vi "PCE-info.vi"(0 "connection ID":refnum<k5>, 11 "error in":errorcluster) -> (4 "connection ID dup":refnum<k5>, 13 "Data Cluster":T1 {"Rotateur" format="%.2f"; "Dome" format="%.2f"; "Focus" format="%.2f"; "Année" format="%.2f"; "Temps Universel" format="%<%H:%M:%S%0u>t"; "Temps Sidéral" format="%<%H:%M:%S%0u>t"; "Masse d'air" format="%.2f"; "Epoque" format="%.2f"; "DEC" format="%<%H:%M:%S%0u>t"; "RA" format="%<%H:%M:%S%0u>t"; "HA" format="%<%H:%M:%S%0u>t"}, 15 "error out":errorcluster)   [LabVIEW 2011]
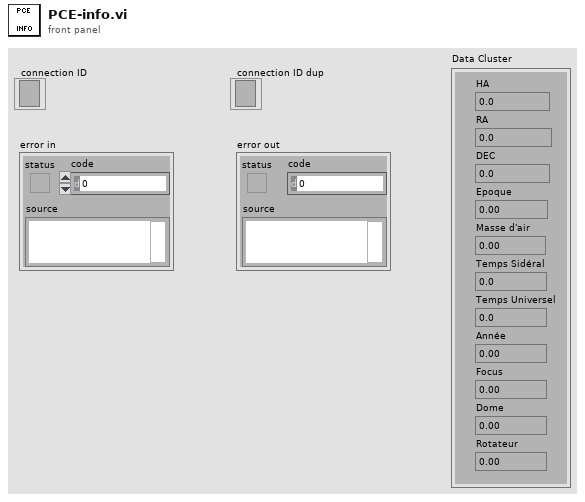
[diagram p1: front panel]
types:
  T1 = cluster{"HA":dbl, "RA":dbl, "DEC":dbl, "Epoque":dbl, "Masse d'air":dbl, "Temps Sidéral":dbl, "Temps Universel":dbl, "Année":dbl, "Focus":dbl, "Dome":dbl, "Rotateur":dbl}
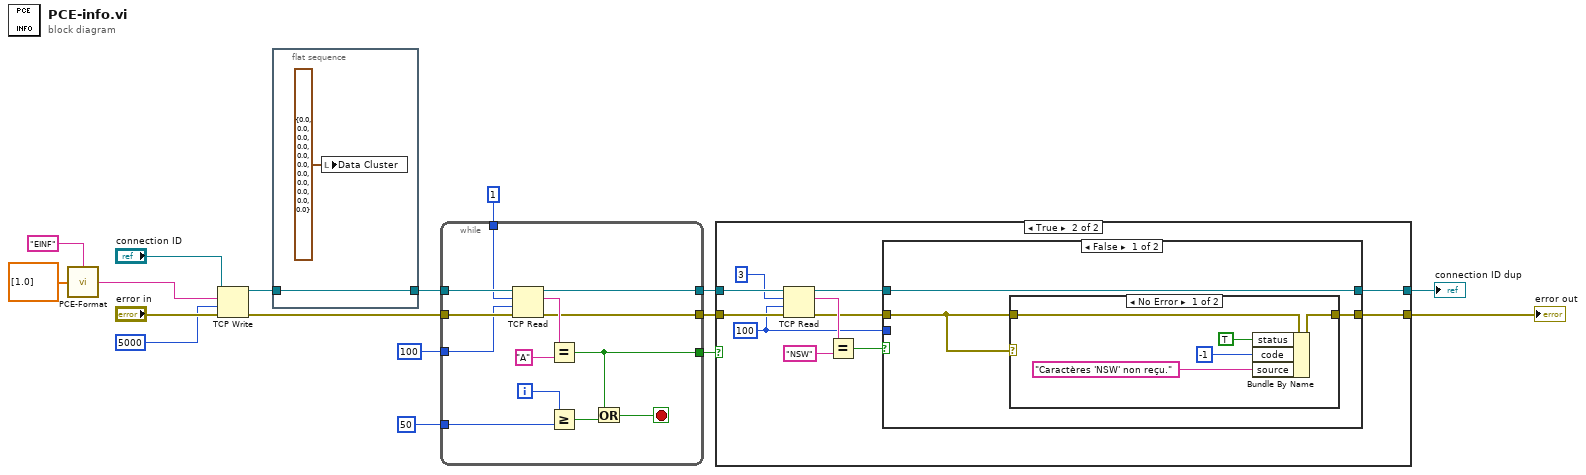
[diagram p0: block diagram]
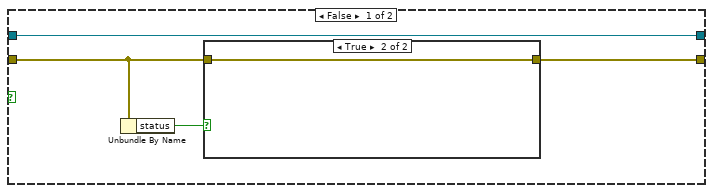
[diagram p2: hidden frame]
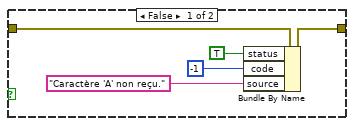
[diagram p3: hidden frame]
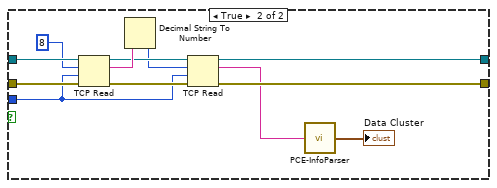
[diagram p5: hidden frame]
diagram:
  n1 = call "PCE-Format.vi"("Commande"="EINF" ("data in"), "Arguments"=dbl[] [1.0]) -> ("Chaîne formatée"=w1:string)  [unwired: 13 in]
  n2 = TCP Write(connection ID="connection ID", data in=w1, error in (no error)="error in", 9:5000 ("timeout ms (25000)")) -> (connection ID out=w5:refnum<k5>, error out=w14:errorcluster)  [unwired: 1 out]
  n3 = flat-sequence {
    tunnel: [w19] -> w4
    tunnel: w5 -> [w19]
    frame #0 {
      n4 = local write "Data Cluster"(T1 {"HA"=0.0, "RA"=0.0, "DEC"=0.0, "Epoque"=0.0, "Masse d'air"=0.0, "Temps Sidéral"=0.0, "Temps Universel"=0.0, "Année"=0.0, "Focus"=0.0, "Dome"=0.0, "Rotateur"=0.0} ("Data Cluster")) -> ()
    }
  }
  n5 = while {
    tunnel: w14 -> [w31]
    tunnel: w4 -> [w32]
    tunnel: [w26] -> w12
    tunnel: [w25] -> w11
    tunnel: [w23] -> w13
    tunnel: 100 ("timeout ms (25000)") -> [w22]
    tunnel: 1 ("bytes to read") -> [w21]
    tunnel: 50 ("y") -> [w20]
    i -> [w30]
    stop <- w24 stop-if-true
    n6 = TCP Read(connection ID=w32, bytes to read=w21, error in (no error)=w31, 9:w22) -> (connection ID out=w25:refnum<k5>, data out=w29:string, error out=w26:errorcluster)  [unwired: 1 in]
    n7 = Equal?(x=w29, y="A") -> (x = y?=w23:bool)
    n8 = Greater Or Equal?(x=w30, y=w20) -> (x >= y?=w27:bool)
    n9 = Or(x=w23, y=w27) -> (x .or. y?=w24:bool)
  }
  n10 = case shown="True" w13 {
    tunnel: w12 -> [w34 w52]
    tunnel: w11 -> [w36 w53]
    tunnel: [w33 w44] -> w7
    tunnel: [w36 w43] -> w6
    frame False {
      n11 = Unbundle By Name(w34) -> ("status"=w35:bool)
      n12 = case shown="True" w35 {
        tunnel: w34 -> [w40 w42]
        tunnel: [w39 w42] -> w33
        frame False {
          n13 = Bundle By Name(cluster=w40, "status"=TRUE, "code"=-1, "source"="Caractère 'A' non reçu.") -> (w39:errorcluster)
        }
        frame True {
        }
      }
    }
    frame True {
      w45 = 100 ("timeout ms (25000)")
      n14 = TCP Read(connection ID=w53, bytes to read=3, error in (no error)=w52, 9:w45) -> (connection ID out=w47:refnum<k5>, data out=w50:string, error out=w46:errorcluster)  [unwired: 1 in]
      n15 = Equal?(x=w50, y="NSW") -> (x = y?=w48:bool)
      n16 = case shown="False" w48 {
        tunnel: w47 -> [w56 w74]
        tunnel: w46 -> [w54 w73]
        tunnel: w45 -> [_ w67]
        tunnel: [w55 w66] -> w44
        tunnel: [w56 w65] -> w43
        frame False {
          n17 = case shown="No Error" w54 {
            tunnel: w54 -> [w60 w62]
            tunnel: [w59 w62] -> w55
            frame No Error {
              n18 = Bundle By Name(cluster=w60, "status"=TRUE, "code"=-1, "source"="Caractères 'NSW' non reçu.") -> (w59:errorcluster)
            }
            frame Error {
            }
          }
        }
        frame True {
          n19 = TCP Read(connection ID=w74, bytes to read=8, error in (no error)=w73, 9:w67) -> (connection ID out=w70:refnum<k5>, data out=w71:string, error out=w69:errorcluster)  [unwired: 1 in]
          n20 = Decimal String To Number(string=w71) -> (number=w68:i32)  [unwired: 2 in, 1 out]
          n21 = TCP Read(connection ID=w70, bytes to read=w68, error in (no error)=w69, 9:w67) -> (connection ID out=w65:refnum<k5>, data out=w64:string, error out=w66:errorcluster)  [unwired: 1 in]
          n22 = call "PCE-InfoParser.vi"("Data String"=w64) -> ("Data Cluster"=→"Data Cluster":T1)  [unwired: 14 in]
        }
      }
    }
  }
  "connection ID dup" <- w6
  "error out" <- w7
